vi "ViewMessageOnMainScreen.vi"(8 "error in (no error)":errorcluster, 11 "Message":T1) -> (0 "error out":errorcluster)   [LabVIEW 2011]
uses:
  030 - EVENTS/03 - ToMessageHandlerProcess/ToMessageHandlerEvent.ctl
  030 - EVENTS/03 - ToMessageHandlerProcess/enumMessageCriticity.ctl
  030 - EVENTS/EnumFgvEventCommand.ctl
  030 - EVENTS/01 - ToHmiScheduler/ToHmiScheduler.ctl
  030 - EVENTS/01 - ToHmiScheduler/ToHmiSchedulerCommand.ctl
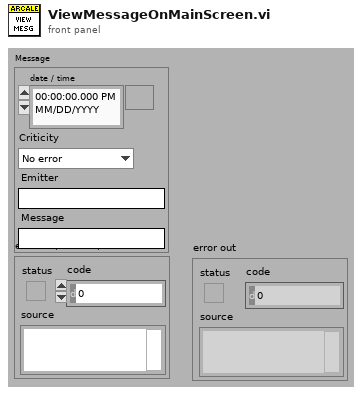
[diagram p1: front panel]
types:
  T1 = typedef "ToMessageHandlerEvent.ctl" = cluster{"date / time":timestamp, "Criticity":T2, "Emitter":string, "Message":string}
  T2 = typedef "enumMessageCriticity.ctl" = enum16{"No error", "Info", "Warning", "Error", "Fatal error"}
  T3 = typedef "ToHmiSchedulerCommand.ctl" = enum16{"Load screen", "Lock screen", "Unlock screen", "Close enable", "Close disable", "Start automatic progress bar", "Stop automatic progress bar", "Set progress bar value (0..100)", "Load previous screen", "Close application", "View message", "Clear message", "Set Window State"}
  T4 = typedef "ToHmiScheduler.ctl" = cluster{"Command":T3, "Screen path":path, "Progress bar value":u8, "Screen Title":string, "To message handler event":T1, "Window_State":enum32{"Invalid", "Standard", "Closed", "Hidden", "Minimized", "Maximized"}}
  T5 = typedef "EnumFgvEventCommand.ctl" = enum16{"Setup", "Cleanup", "Get"}
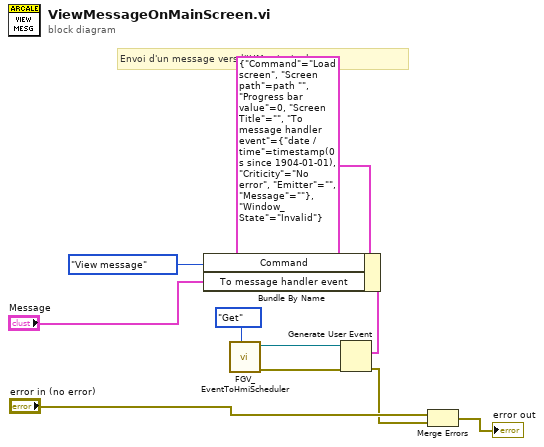
[diagram p0: block diagram]
diagram:
  # "Envoi d'un message vers l'IHM principale ...."
  n1 = Bundle By Name(cluster=T4 {"Command"=enum."Load screen", "Screen path"=path "", "Progress bar value"=0, "Screen Title"="", "To message handler event"={"date / time"=timestamp(0 s since 1904-01-01), "Criticity"=enum."No error", "Emitter"="", "Message"=""}, "Window_State"=enum."Invalid"} ("event data"), "Command"=ToHmiSchedulerCommand."View message", "To message handler event"="Message") -> (w6:T4)
  n2 = call "FGV_EventToHmiScheduler.vi"("Command"=EnumFgvEventCommand."Get") -> ("error out"=w9:errorcluster, "ToHmiSchedulerEvent"=w8:refnum<user-event>)  [unwired: 9 in]
  n3 = Generate User Event(user event=w8, event data cluster=w6, error in=w9) -> (error out=w4:errorcluster)  [unwired: 1 out]
  n4 = Merge Errors("error in (no error)", w4) -> (→"error out":errorcluster)
